vi "RILIS Narrow Band Scan Coordinator 2.0.vi"() -> ()   [LabVIEW 2013]
uses:
  RILIS Narrow Band Scan Coordinator States.ctl
panel:
  out "Waveform Chart":T1(graph)
  in  "RILIS Cancel Button":bool
  in  "Setpoint Reached Thresold":dbl=0.003
  in  "Max Allowed Scan Step (cm-1)":dbl=0.02 format="%.4f"
  out "isNew":bool
  out "waveReadback":dbl format="%#.4f"
  out "waveSet":dbl format="%.4f"
  out "Current State":T2
  out "Actual Wavenumber":dbl format="%#.4f"
  out "Loop Counter":i32
  in  "Stop Program":bool
  out "Measurement Complete":bool
  out "isOK":bool
  out "Linewidth Sweep Done":bool
  out "Moving to Setpoint":bool
  out "Setpoint Wavenumber":dbl format="%.4f"
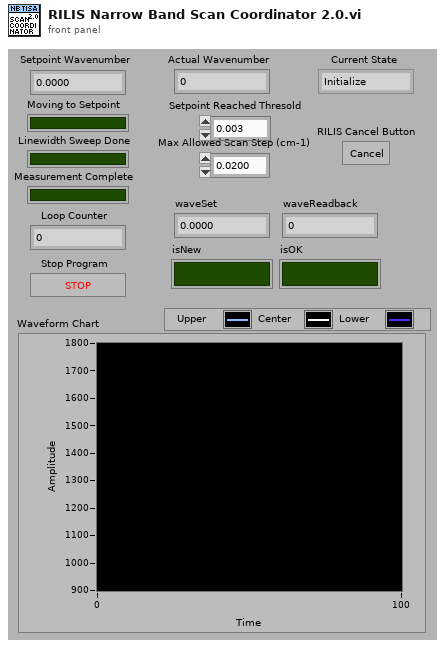
[diagram p1: front panel]
types:
  T1 = cluster{"Upper Limit":i32, "Center Position":i32, "Lower Limit":i32}
  T2 = typedef "RILIS Narrow Band Scan Coordinator States.ctl" = enum16{"Initialize", "Idle", "Read Setpoint WN", "Check Setpoint WN", "Move to Setpoint WN", "Perform Sweep", "Wait for Ready", "Measurement in Progress", "Stop"}
  T3 = cluster{"Moving to Setpoint":bool, "Linewidth Sweep Done":bool, "Ready to Average":bool, "Averaging Active":bool, "Measurement Complete":bool, "Setpoint Wavenumber":dbl}
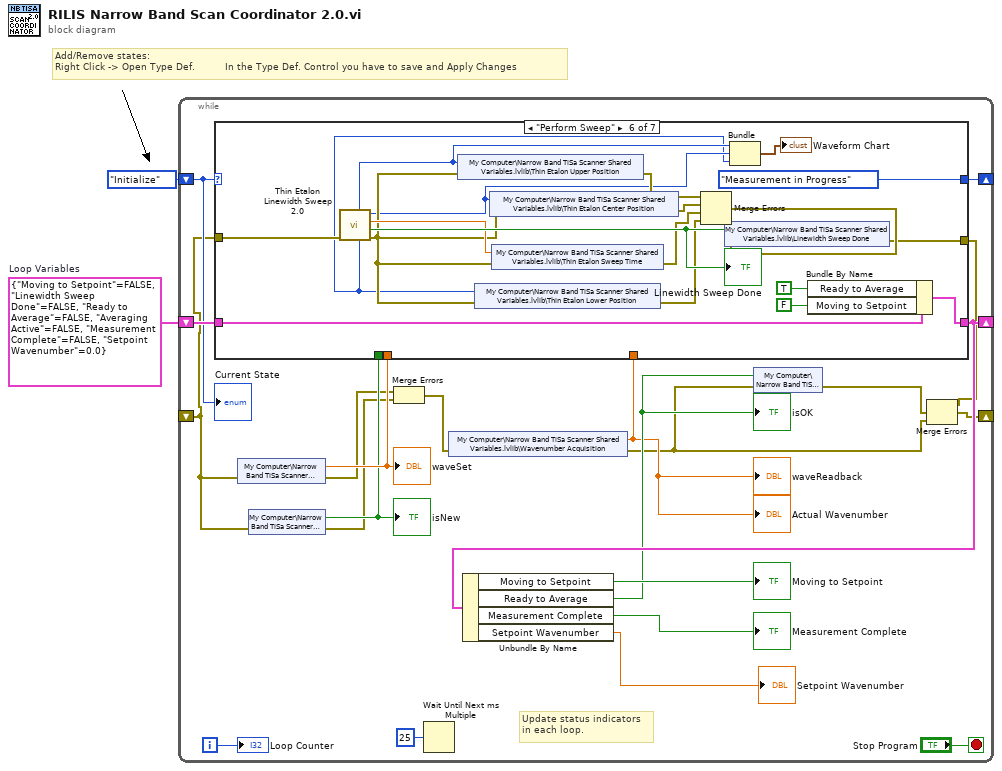
[diagram p0: block diagram]
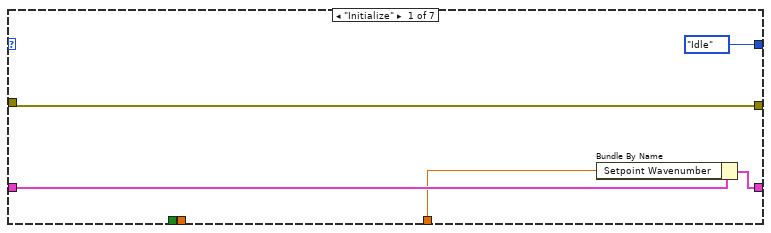
[diagram p2: hidden frame]
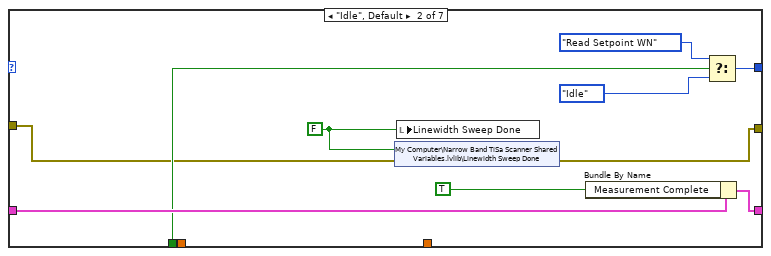
[diagram p3: hidden frame]
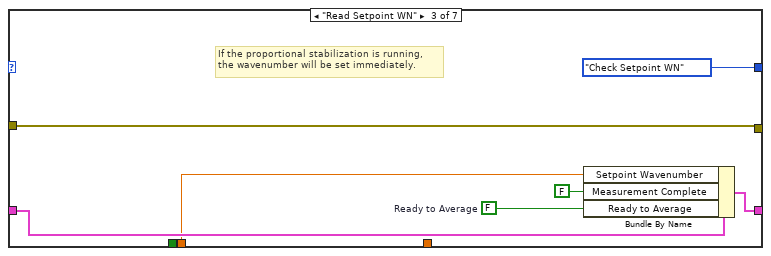
[diagram p4: hidden frame]
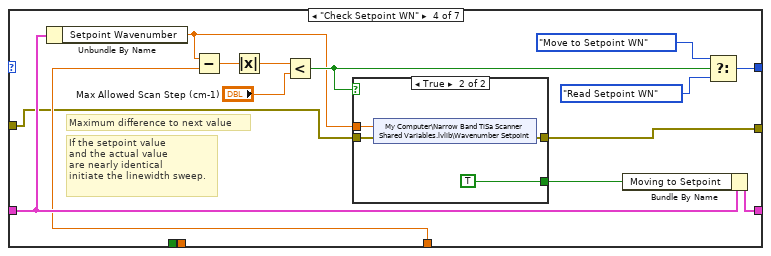
[diagram p5: hidden frame]
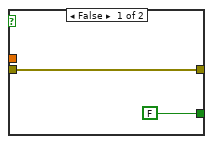
[diagram p6: hidden frame]
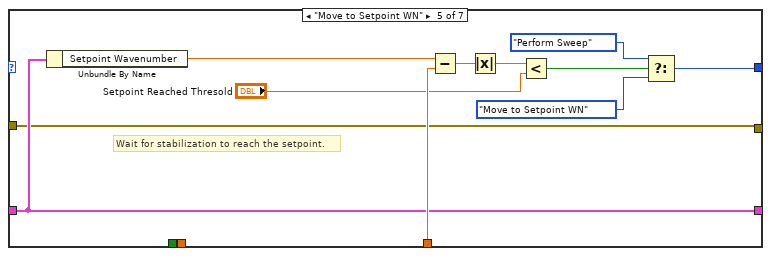
[diagram p7: hidden frame]
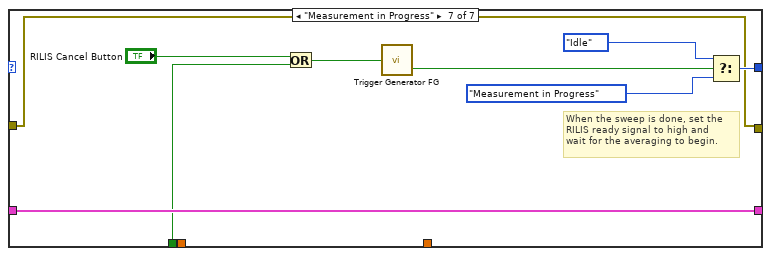
[diagram p8: hidden frame]
diagram:
  w1 = T3 {"Moving to Setpoint"=FALSE, "Linewidth Sweep Done"=FALSE, "Ready to Average"=FALSE, "Averaging Active"=FALSE, "Measurement Complete"=FALSE, "Setpoint Wavenumber"=0.0}  # Loop Variables
  # "Add/Remove states:\nRight Click -> Open Type Def.          In the Type Def. Control you have to save and Apply Changes"
  n1 = while {
    shift-right: [w21] -> _
    shift-left: RILIS_Narrow_Band_Scan_Coordinator_States."Initialize" ("NB Scan States") -> [w19]
    shift-right: [w18] -> _
    shift-left: w1 -> [w20]
    shift-right: [w8] -> _
    shift-left: _ -> [w4]
    i -> [w23]
    stop <- "Stop Program" stop-if-true
    # "Update status indicators \nin each loop."
    n2 = shared-variable "My Computer\\Narrow Band TiSa Scanner Shared Variables.lvlib\\waveSet"(error in=w4) -> (w14:dbl, error out=w11:errorcluster)
    "waveSet" <- w14
    n3 = shared-variable "My Computer\\Narrow Band TiSa Scanner Shared Variables.lvlib\\isNew"(error in=w4) -> (w13:bool, error out=w10:errorcluster)
    "isNew" <- w13
    n4 = Merge Errors(w11, w10) -> (w9:errorcluster)
    n5 = Wait Until Next ms Multiple(millisecond multiple=u32 25) -> ()  [unwired: 1 out]
    n6 = shared-variable "My Computer\\Narrow Band TiSa Scanner Shared Variables.lvlib\\Wavenumber Acquisition"(error in=w9) -> (w7:dbl, error out=w3:errorcluster)
    "Actual Wavenumber" <- w7
    "waveReadback" <- w7
    n7 = case shown="\"Perform Sweep\"" w19 {
      tunnel: [RILIS_Narrow_Band_Scan_Coordinator_States."Idle" ("NB Scan States") w37 RILIS_Narrow_Band_Scan_Coordinator_States."Check Setpoint WN" ("NB Scan States") w55 w68 RILIS_Narrow_Band_Scan_Coordinator_States."Measurement in Progress" ("NB Scan States") w103] -> w21
      tunnel: w20 -> [w28 w35 w45 w53 w74 w94 w101]
      tunnel: [w27 w34 w44 w54 w74 w93 w101] -> w18
      tunnel: w13 -> [_ w33 _ _ _ _ w100]
      tunnel: w14 -> [_ _ w43 _ _ _ _]
      tunnel: w7 -> [w26 _ _ w52 w75 _ _]
      tunnel: [w25 w30 w40 w47 w67 w83 w97] -> w5
      tunnel: w4 -> [w25 w31 w40 w48 w67 w82 w97]
      frame "Initialize" {
        n8 = Bundle By Name(cluster=w28, "Setpoint Wavenumber"=w26) -> (w27:T3)
      }
      frame "Idle", Default {
        w32 = FALSE
        n9 = shared-variable "My Computer\\Narrow Band TiSa Scanner Shared Variables.lvlib\\Linewidth Sweep Done"(w32, error in=w31) -> (error out=w30:errorcluster)
        n10 = local write "Linewidth Sweep Done"(w32) -> ()
        n11 = Bundle By Name(cluster=w35, "Measurement Complete"=TRUE) -> (w34:T3)
        n12 = Select(t=RILIS_Narrow_Band_Scan_Coordinator_States."Read Setpoint WN" ("NB Scan States"), s=w33, f=RILIS_Narrow_Band_Scan_Coordinator_States."Idle" ("NB Scan States")) -> (s? t:f=w37:T2)
      }
      frame "Read Setpoint WN" {
        w42 = FALSE  # Ready to Average
        # "If the proportional stabilization is running, \nthe wavenumber will be set immediately."
        n13 = Bundle By Name(cluster=w45, "Setpoint Wavenumber"=w43, "Measurement Complete"=FALSE, "Ready to Average"=w42) -> (w44:T3)
      }
      frame "Check Setpoint WN" {
        # "Maximum difference to next value"
        # "If the setpoint value \nand the actual value\nare nearly identical \ninitiate the linewidth sweep."
        n14 = Unbundle By Name(w53) -> ("Setpoint Wavenumber"=w50:dbl)
        n15 = Subtract(x=w50, y=w52) -> (x-y=w60:dbl)
        n16 = Absolute Value(x=w60) -> (abs(x)=w59:dbl)
        n17 = Less?(x=w59, y="Max Allowed Scan Step (cm-1)") -> (x < y?=w51:bool)
        n18 = case shown="True" w51 {
          tunnel: w50 -> [_ w66]
          tunnel: [FALSE TRUE] -> w49
          tunnel: w48 -> [w61 w64]
          tunnel: [w61 w63] -> w47
          frame False {
          }
          frame True {
            n19 = shared-variable "My Computer\\Narrow Band TiSa Scanner Shared Variables.lvlib\\Wavenumber Setpoint"(w66, error in=w64) -> (error out=w63:errorcluster)
          }
        }
        n20 = Bundle By Name(cluster=w53, "Moving to Setpoint"=w49) -> (w54:T3)
        n21 = Select(t=RILIS_Narrow_Band_Scan_Coordinator_States."Move to Setpoint WN" ("NB Scan States"), s=w51, f=RILIS_Narrow_Band_Scan_Coordinator_States."Read Setpoint WN" ("NB Scan States")) -> (s? t:f=w55:T2)
      }
      frame "Move to Setpoint WN" {
        # "Wait for stabilization to reach the setpoint."
        n22 = Unbundle By Name(w74) -> ("Setpoint Wavenumber"=w73:dbl)
        n23 = Subtract(x=w73, y=w75) -> (x-y=w77:dbl)
        n24 = Absolute Value(x=w77) -> (abs(x)=w76:dbl)
        n25 = Less?(x=w76, y="Setpoint Reached Thresold") -> (x < y?=w71:bool)
        n26 = Select(t=RILIS_Narrow_Band_Scan_Coordinator_States."Perform Sweep" ("NB Scan States"), s=w71, f=RILIS_Narrow_Band_Scan_Coordinator_States."Move to Setpoint WN" ("NB Scan States")) -> (s? t:f=w68:T2)
      }
      frame "Perform Sweep" {
        n27 = call "Thin Etalon Linewidth Sweep 2.0.vi"("Error In"=w82) -> ("Error Out"=w89:errorcluster, "Done"=w92:bool, "Time Elapsed"=w90:dbl, "Center Position"=w80:i32, "Lower Limit"=w79:i32, "Upper Limit"=w81:i32)  [unwired: 5 in]
        "Linewidth Sweep Done" <- w92
        n28 = shared-variable "My Computer\\Narrow Band TiSa Scanner Shared Variables.lvlib\\Thin Etalon Upper Position"(w81, error in=w89) -> (error out=w88:errorcluster)
        n29 = shared-variable "My Computer\\Narrow Band TiSa Scanner Shared Variables.lvlib\\Thin Etalon Lower Position"(w79, error in=w89) -> (error out=w84:errorcluster)
        n30 = shared-variable "My Computer\\Narrow Band TiSa Scanner Shared Variables.lvlib\\Thin Etalon Center Position"(w80, error in=w89) -> (error out=w87:errorcluster)
        n31 = shared-variable "My Computer\\Narrow Band TiSa Scanner Shared Variables.lvlib\\Thin Etalon Sweep Time"(w90, error in=w89) -> (error out=w85:errorcluster)
        n32 = Merge Errors(w88, w87, w85, w84) -> (w86:errorcluster)
        n33 = shared-variable "My Computer\\Narrow Band TiSa Scanner Shared Variables.lvlib\\Linewidth Sweep Done"(w92, error in=w86) -> (error out=w83:errorcluster)
        n34 = Bundle("Upper Limit"=w81, "Center Position"=w80, "Lower Limit"=w79) -> (→"Waveform Chart":T1)  [unwired: 1 in]
        n35 = Bundle By Name(cluster=w94, "Ready to Average"=TRUE, "Moving to Setpoint"=FALSE) -> (w93:T3)
      }
      frame "Measurement in Progress" {
        # "When the sweep is done, set the \nRILIS ready signal to high and \nwait for the averaging to begin."
        n36 = Or(x="RILIS Cancel Button", y=w100) -> (x .or. y?=w99:bool)
        n37 = call "Trigger Generator FG.vi"("Boolean in"=w99) -> ("Falling Trigger out"=w102:bool)  [unwired: 1 out]
        n38 = Select(t=RILIS_Narrow_Band_Scan_Coordinator_States."Idle" ("NB Scan States"), s=w102, f=RILIS_Narrow_Band_Scan_Coordinator_States."Measurement in Progress" ("NB Scan States")) -> (s? t:f=w103:T2)
      }
    }
    n39 = Unbundle By Name(w18) -> ("Moving to Setpoint"=→"Moving to Setpoint":bool, "Ready to Average"=w15:bool, "Measurement Complete"=→"Measurement Complete":bool, "Setpoint Wavenumber"=→"Setpoint Wavenumber":dbl)
    "isOK" <- w15
    n40 = shared-variable "My Computer\\Narrow Band TiSa Scanner Shared Variables.lvlib\\isOK"(w15, error in=w3) -> (error out=w12:errorcluster)
    n41 = Merge Errors(w5, w12, w3) -> (w8:errorcluster)
    "Loop Counter" <- w23
    "Current State" <- w19
  }
